vi "encodeMessage.vi"(8 "error in (no error)":errorcluster, 10 "Data in":refnum<class>, 11 "CameraNetworkClient in":refnum<class "CameraNetworkServer.lvclass">) -> (0 "error out":errorcluster, 2 "messageString":string, 3 "CameraNetworkClient out":refnum<class "CameraNetworkServer.lvclass">)   [LabVIEW 2011, in "Hardware.lvlib" / "HWControllers.lvlib" / "CameraNetworkServer.lvclass"]
uses:
  CameraNetworkServer.lvclass
  NetworkClient/NetworkServer.lvclass
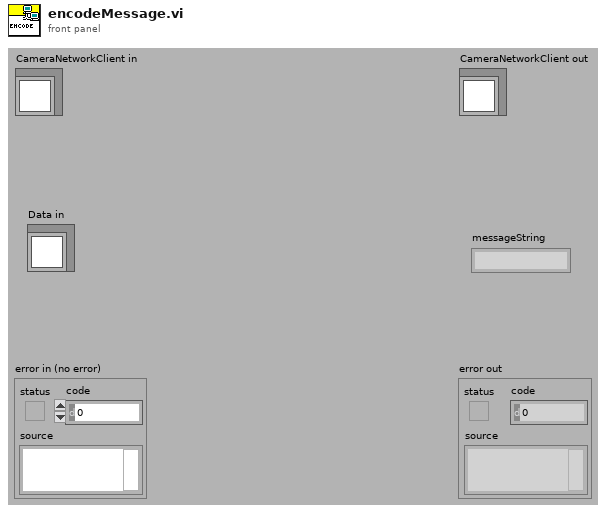
[diagram p1: front panel]
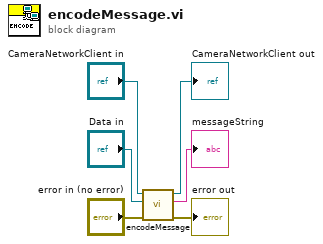
[diagram p0: block diagram]
diagram:
  n1 = call-parent "encodeMessage.vi"("error in (no error)"="error in (no error)", "Data in"="Data in", "NetworkClient in"="CameraNetworkClient in") -> ("error out"=→"error out":errorcluster, "messageString"=→"messageString":string, "NetworkClient out"=→"CameraNetworkClient out":refnum<class "CameraNetworkServer.lvclass">)  [unwired: 6 in]
